vi "Length_8.vi"() -> ()   [LabVIEW 2020]
uses:
  Support/Controls/Cmd_Mouse Popup.ctl
  Support/Controls/Clst_Initialize Input.ctl
  Support/Controls/Clst_Result inspec.ctl
  Support/Controls/Cmd_Var Data IO.ctl
  Variables/Global_Cal Info.vi
  Variables/Global_Cal STD.vi
  Support/Public/Polymorph/Data Class_2D Str.vi
panel:
  in  "기준기 설정":string(combo)
  out "최소범위":string
  out "STD set":string[][](table) caption="○ 기준기 조합 (값)"
  in  "Measured 2":string[][](table)
  in  "표시방식":string(combo)
  out "단위":string
  out "최대범위":string
  in  "Spec 변경":bool
  in  "Random":bool
  out "Resolution":string[][](table) caption="Spec"
  out "Spec":string[][](table)
  out "제목":string
  out "에러 출력":errorcluster
  out "Condition":string[][](table) caption="2. 직선성 시험"
  in  "최소눈금":string(combo)
  in  "Measured":string[][](table) caption="지시편차 (μm)"
  out "Load?":bool
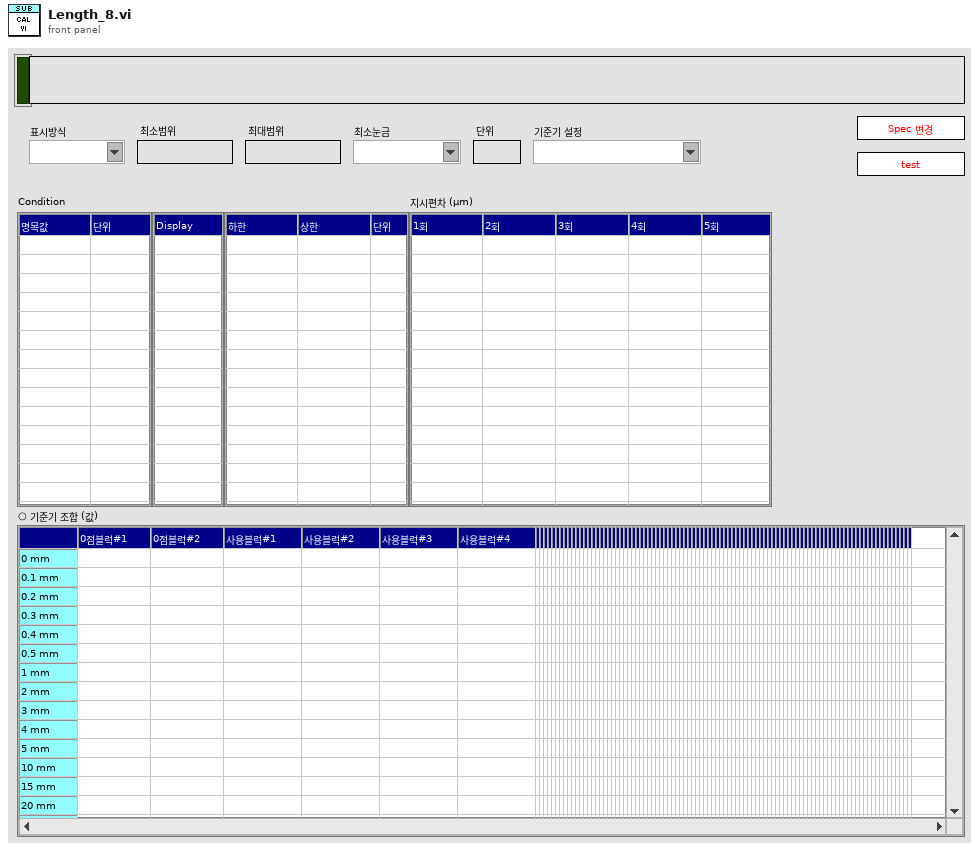
[diagram p1: front panel]
types:
  T1 = typedef "Cmd_Mouse Popup.ctl" = enum16{"활성화", "메뉴선택"}
  T2 = cluster{"Shift":bool, "Ctrl":bool, "Alt":bool, "Cmd":bool, "Opt":bool}
  T3 = typedef "Clst_Initialize Input.ctl" = cluster{"Initialize 1":cluster{"Condition":refnum<vi>[], "Spec":refnum<vi>[], "Measured":refnum<vi>[], "Resolution":refnum<vi>[], "Func_ext":string, "제목":refnum<vi>, "Measured_ADJ":refnum<vi>[]}, "Initialize 2":cluster{"문자열":refnum<vi>[], "콤보박스":refnum<vi>[], "링":refnum<vi>[], "열거형":refnum<vi>[], "테이블":refnum<vi>[], "여러열":refnum<vi>[], "디지털(DBL)":refnum<vi>[], "3D string":refnum<vi>[], "ctrl":refnum<vi>[], "boolean":refnum<vi>[]}}
  T4 = typedef "Clst_Result inspec.ctl" = cluster{"분해능":string, "문자열 1":string, "문자열 2":string, "숫자형 1":i32, "숫자형 2":i32, "숫자형 3":dbl, "문자배열 1D":string[], "문자배열 2D":string[][], "문자배열 3D":string[][][], "문자배열 4D":string[][][][], "불리언 1D":bool[]}
  T5 = typedef "Cmd_Var Data IO.ctl" = enum16{"Condition", "Condition Default", "Condition_Temp", "Resolution", "Resolution Default", "Resolution Old", "Spec", "Spec Default", "Spec Old", "Spec Temp", "Result", "Result2", "Result3", "Result_Temp", "Result_ADJ", "Result_ADJ2", "STD1", "STD2", "STD3", "STD4", "STD5", "STD Temp", "CMC", "CMC Default"}
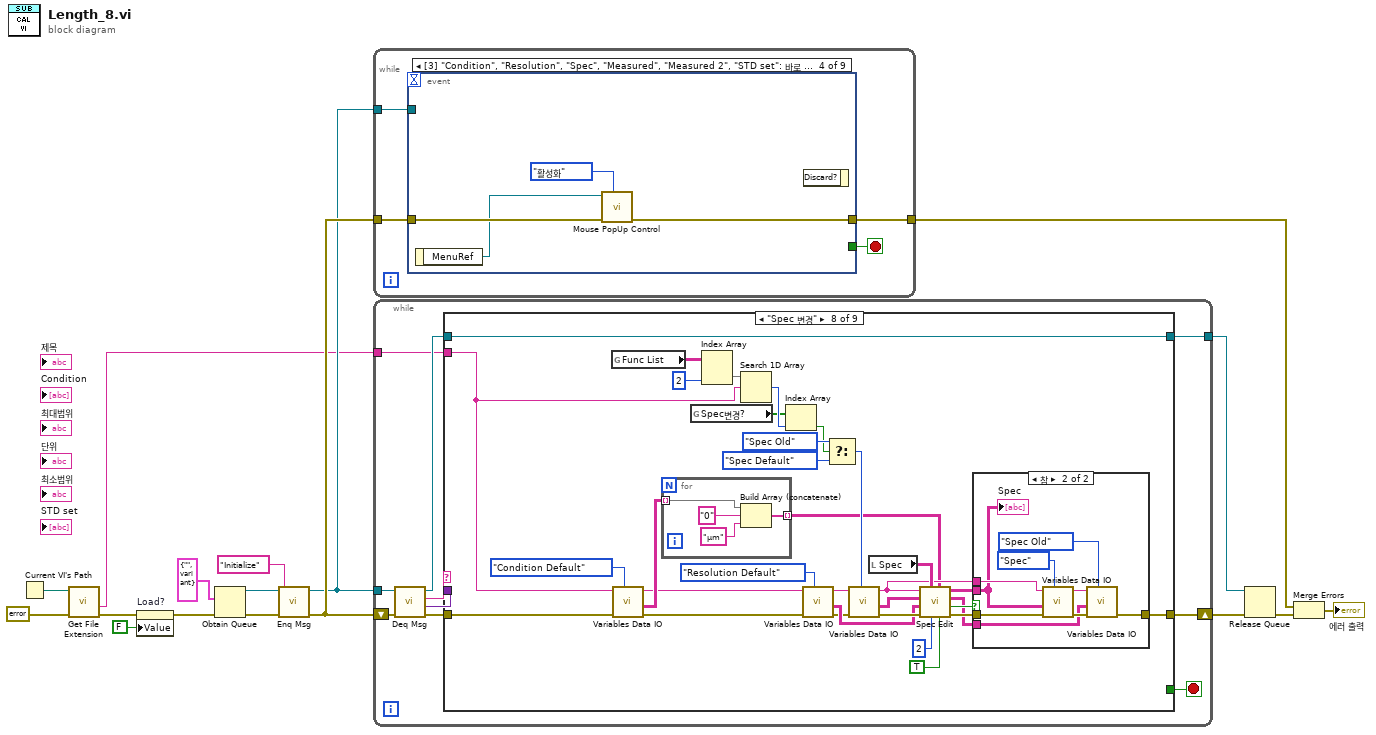
[diagram p0: block diagram]
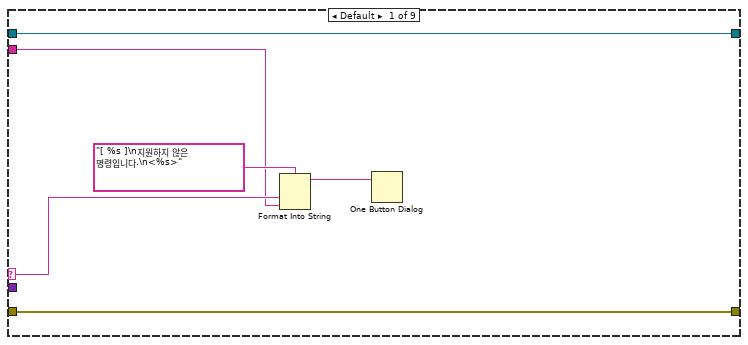
[diagram p2: hidden frame]
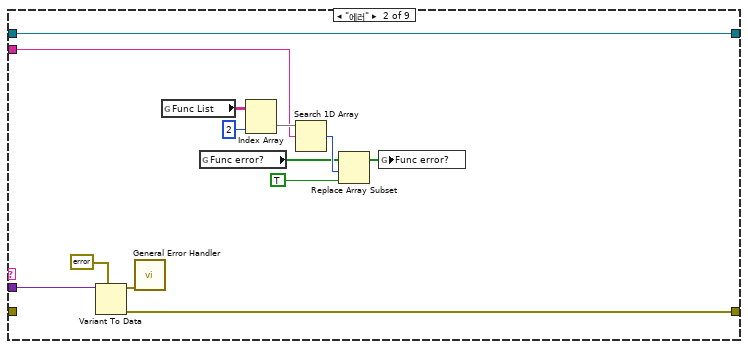
[diagram p3: hidden frame]
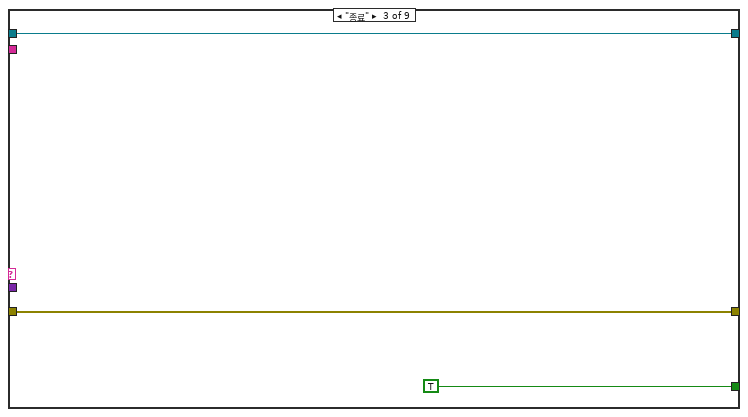
[diagram p4: hidden frame]
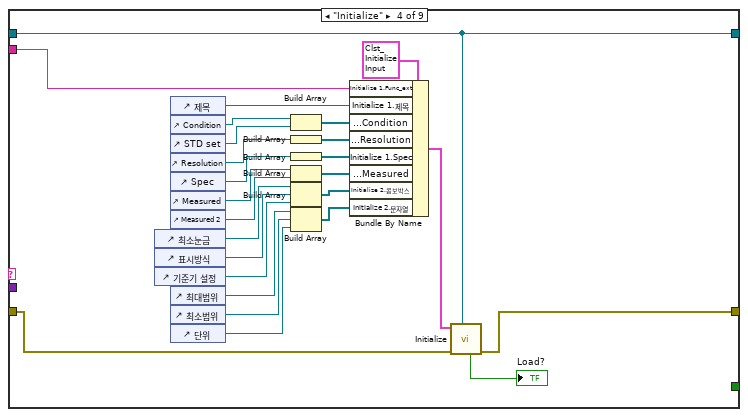
[diagram p5: hidden frame]
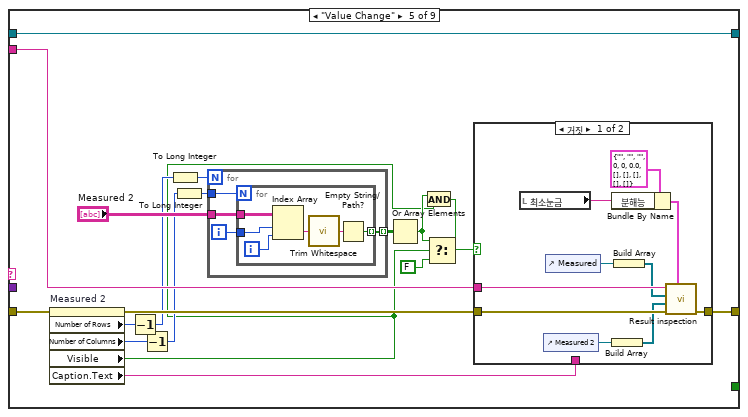
[diagram p6: hidden frame]
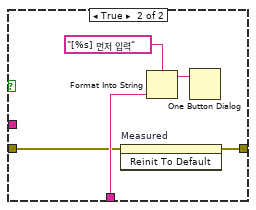
[diagram p7: hidden frame]
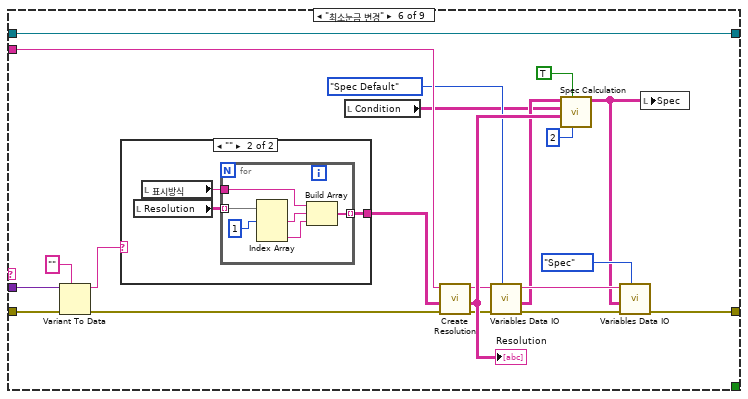
[diagram p8: hidden frame]
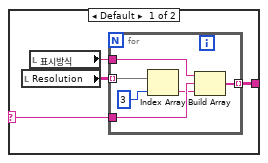
[diagram p9: hidden frame]
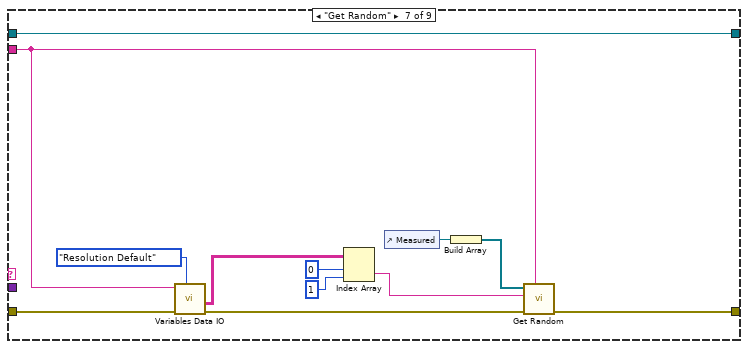
[diagram p10: hidden frame]
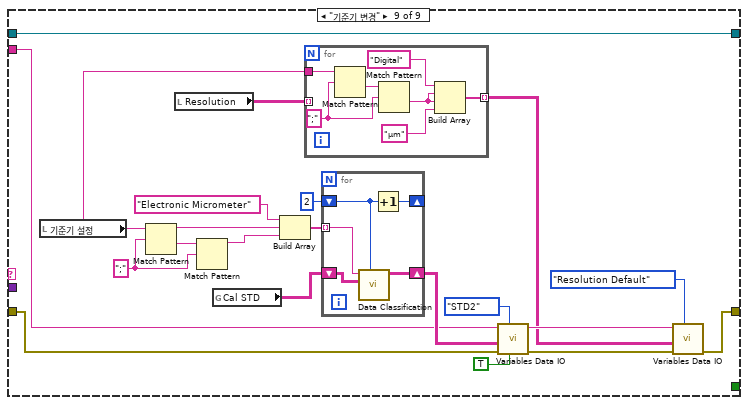
[diagram p12: hidden frame]
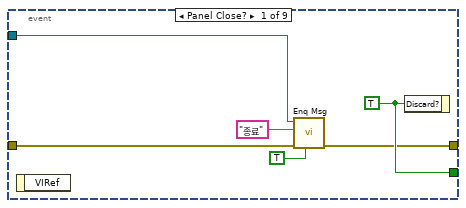
[diagram p13: hidden frame]
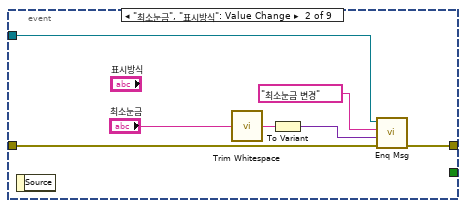
[diagram p14: hidden frame]
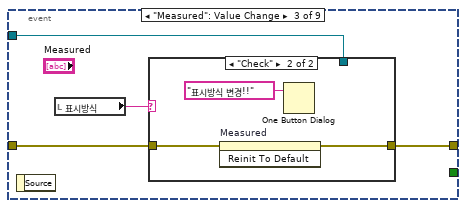
[diagram p15: hidden frame]
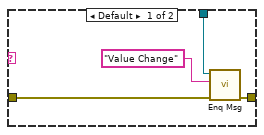
[diagram p16: hidden frame]
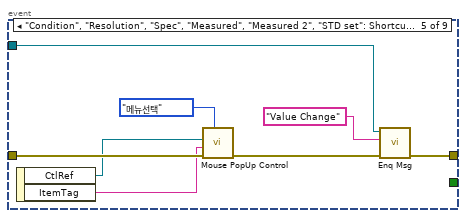
[diagram p17: hidden frame]
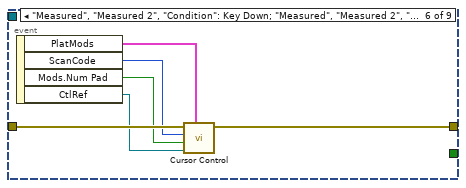
[diagram p18: hidden frame]
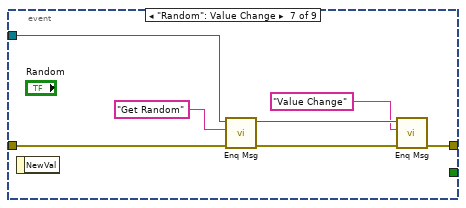
[diagram p19: hidden frame]
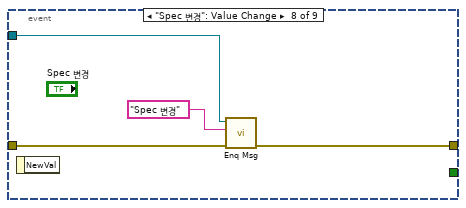
[diagram p20: hidden frame]
diagram:
  n1 = Current VI's Path() -> (path=w5:path)
  n2 = call <vilib>:"Get File Extension.vi"("error in (no error)"=errorcluster {"status"=FALSE, "code"=0, "source"=""} ("에러 상수"), "file"=w5) -> ("error out"=w3:errorcluster, "filename without extension"=w4:string)  [unwired: 5 in, 3 out]
  n3 = property on="Load?" class="Bool (엄격한)"(error in=w3, "Value"=FALSE ("Load?")) -> (error out=w2:errorcluster)  [unwired: 1 in, 1 out]
  n4 = Obtain Queue(element data type=cluster{"메세지":string, "값":variant} {"메세지"="", "값"=variant} ("Message Cluster"), error in (no error)=w2) -> (queue out=w14:refnum<queue>, error out=w16:errorcluster)  [unwired: 3 in, 1 out]
  n5 = call "Enq Msg.vi"("에러 입력(에러 없음)"=w16, "메세지"="Initialize", "큐 입력"=w14) -> ("에러 출력"=w15:errorcluster, "큐 출력"=w12:refnum<queue>)  [unwired: 7 in]
  n6 = while {
    tunnel: w15 -> [w19]
    tunnel: w12 -> [w20]
    tunnel: [w18] -> w9
    stop <- w21 stop-if-true
    n7 = event shown="[3] \"Condition\", \"Resolution\", \"Spec\", \"Measured\", \"Measured 2\", \"STD set\": 바로 가기 메뉴 활성화?" {
      selector: _ -> [_ _ _ _ _ _ _ _ _]
      dyn-events: _ -> [_ _ _ _ _ _ _ _ _]
      timeout: _ -> [_ _ _ _ _ _ _ _ _]
      tunnel: [w27 _ _ _ _ _ _ _ _] -> w21
      tunnel: w20 -> [w25 w33 w38 _ w50 _ w68 w72 w75]
      tunnel: w19 -> [w26 w34 w36 w49 w57 w63 w69 w73 w77]
      tunnel: [w23 w32 w37 w48 w51 w62 w64 w71 w76] -> w18
      event Panel Close? {
        w27 = TRUE ("버림?")
        n8 = event-data() -> ()  [unwired: 1 in, 1 out]
        n9 = call "Enq Msg.vi"("우선순위 메시지?"=TRUE, "에러 입력(에러 없음)"=w26, "메세지"="종료", "큐 입력"=w25) -> ("에러 출력"=w23:errorcluster)  [unwired: 6 in, 1 out]
        n10 = event-data("Discard?"=w27) -> ()  [unwired: 1 in, 1 out]
      }
      event "최소눈금", "표시방식": Value Change {
        n11 = event-data() -> ()  [unwired: 1 in, 1 out]
        n12 = call <vilib>:"Trim Whitespace.vi"("string"="최소눈금") -> ("trimmed string"=w30:string)  [unwired: 1 in]
        n13 = To Variant(anything=w30) -> (Variant=w28:variant)
        n14 = call "Enq Msg.vi"("에러 입력(에러 없음)"=w34, "값"=w28, "메세지"="최소눈금 변경", "큐 입력"=w33) -> ("에러 출력"=w32:errorcluster)  [unwired: 6 in, 1 out]
      }
      event "Measured": Value Change {
        n15 = event-data() -> ()  [unwired: 1 in, 1 out]
        n16 = local read "표시방식"() -> (w35:string)
        n17 = case shown="\"Check\"" w35 {
          tunnel: w38 -> [w42 _]
          tunnel: [w41 w43] -> w37
          tunnel: w36 -> [w40 w44]
          frame Default {
            n18 = call "Enq Msg.vi"("에러 입력(에러 없음)"=w40, "메세지"="Value Change", "큐 입력"=w42) -> ("에러 출력"=w41:errorcluster)  [unwired: 7 in, 1 out]
          }
          frame "Check" {
            n19 = invoke on="Measured" class="Tbl (엄격한)" method="Reinit To Default"(error in=w44) -> (error out=w43:errorcluster)  [unwired: 2 in, 2 out]
            n20 = One Button Dialog(message="표시방식 변경!!" ("메시지")) -> ()  [unwired: 1 in, 1 out]
          }
        }
      }
      event "Condition", "Resolution", "Spec", "Measured", "Measured 2", "STD set": Shortcut Menu Activation? {
        n21 = event-data() -> ("MenuRef"=w47:refnum<k9>)  [unwired: 1 in]
        n22 = call "Mouse PopUp Control.vi"("type"=Cmd_Mouse_Popup."활성화", "error in"=w49, "메뉴 참조"=w47) -> ("error out"=w48:errorcluster)  [unwired: 8 in]
        n23 = event-data() -> ()  [unwired: 2 in, 1 out]
      }
      event "Condition", "Resolution", "Spec", "Measured", "Measured 2", "STD set": Shortcut Menu Selection (User) {
        n24 = event-data() -> ("CtlRef"=w55:refnum<vi>, "ItemTag"=w54:string)  [unwired: 1 in]
        n25 = call "Mouse PopUp Control.vi"("type"=Cmd_Mouse_Popup."메뉴선택", "error in"=w57, "아이템 태그"=w54, "Tbl 참조 번호"=w55) -> ("error out"=w52:errorcluster)  [unwired: 7 in]
        n26 = call "Enq Msg.vi"("에러 입력(에러 없음)"=w52, "메세지"="Value Change", "큐 입력"=w50) -> ("에러 출력"=w51:errorcluster)  [unwired: 7 in, 1 out]
      }
      event "Measured", "Measured 2", "Condition": Key Down; "Measured", "Measured 2", "Condition": Key Repeat {
        n27 = event-data() -> ("PlatMods"=w58:T2, "ScanCode"=w61:i16, "Mods.Num Pad"=w60:bool, "CtlRef"=w59:refnum<vi>)  [unwired: 1 in]
        n28 = call "Cursor Control.vi"("플랫폼 조합키"=w58, "참조"=w59, "Num Pad"=w60, "ScanCode"=w61, "error in"=w63) -> ("error out"=w62:errorcluster)  [unwired: 5 in, 1 out]
      }
      event "Random": Value Change {
        n29 = event-data() -> ()  [unwired: 1 in, 1 out]
        n30 = call "Enq Msg.vi"("에러 입력(에러 없음)"=w69, "메세지"="Get Random", "큐 입력"=w68) -> ("에러 출력"=w67:errorcluster, "큐 출력"=w66:refnum<queue>)  [unwired: 7 in]
        n31 = call "Enq Msg.vi"("에러 입력(에러 없음)"=w67, "메세지"="Value Change", "큐 입력"=w66) -> ("에러 출력"=w64:errorcluster)  [unwired: 7 in, 1 out]
      }
      event "Spec 변경": Value Change {
        n32 = event-data() -> ()  [unwired: 1 in, 1 out]
        n33 = call "Enq Msg.vi"("에러 입력(에러 없음)"=w73, "메세지"="Spec 변경", "큐 입력"=w72) -> ("에러 출력"=w71:errorcluster)  [unwired: 7 in, 1 out]
      }
      event "기준기 설정": Value Change {
        n34 = event-data() -> ()  [unwired: 1 in, 2 out]
        n35 = call "Enq Msg.vi"("에러 입력(에러 없음)"=w77, "메세지"="기준기 변경", "큐 입력"=w75) -> ("에러 출력"=w76:errorcluster)  [unwired: 7 in, 1 out]
      }
    }
  }
  n36 = while {
    shift-right: [w88] -> w11
    shift-left: w15 -> [w87]
    tunnel: w12 -> [w85]
    tunnel: [w80] -> w10
    tunnel: w4 -> [w79]
    stop <- w81 stop-if-true
    n37 = call "Deq Msg.vi"("에러 입력(에러 없음)"=w87, "큐 입력"=w85) -> ("에러 출력"=w86:errorcluster, "값"=w82:variant, "메세지"=w84:string, "큐 출력"=w83:refnum<queue>)  [unwired: 6 in]
    n38 = case shown="\"Spec 변경\"" w84 {
      selector: w84 -> [w90 _ _ _ _ _ _ _ _]
      tunnel: w86 -> [w94 _ w110 w113 w150 w199 w227 w239 w291]
      tunnel: [w94 w104 w110 w127 w153 w192 w228 w259 w286] -> w88
      tunnel: w83 -> [w93 w103 w108 w121 w154 w200 w231 w263 w298]
      tunnel: w82 -> [_ w105 _ _ _ w198 _ _ _]
      tunnel: [_ _ TRUE ("버림?") _ _ _ _ _ _] -> w81
      tunnel: [w93 w103 w108 w121 w154 w200 w231 w263 w298] -> w80
      tunnel: w79 -> [w89 w95 _ w122 w152 w196 w224 w233 w290]
      frame Default {
        n39 = Format Into String(format string="[ %s ]\n지원하지 않은 명령입니다.\n<%s>" ("메시지"), w90, w89) -> (resulting string=w91:string)  [unwired: 2 in, 1 out]
        n40 = One Button Dialog(message=w91) -> ()  [unwired: 1 in, 1 out]
      }
      frame "에러" {
        n41 = Variant To Data(type=errorcluster {"status"=FALSE, "code"=0, "source"=""} ("에러 출력"), Variant=w105) -> (data=w107:errorcluster, error out=w104:errorcluster)  [unwired: 1 in]
        n42 = call <vilib>:"General Error Handler.vi"("error in (no error)"=w107) -> ()  [unwired: 10 in, 5 out]
        n43 = global read "Global_Cal Info.vi" "Func List"() -> (w97:string[][])
        n44 = global read "Global_Cal Info.vi" "Func error?"() -> (w100:bool[])
        n45 = Index Array(array=w97, index (col)=2 ("비활성화된 인덱스 (열)")) -> (element=w98:string[])  [unwired: 1 in]
        n46 = Search 1D Array(1D array=w98, element=w95) -> (index of element=w101:i32)  [unwired: 1 in]
        n47 = Replace Array Subset(array=w100, new element=TRUE ("새 원소/부분배열"), index=w101) -> (w102:bool[])
        n48 = global write "Global_Cal Info.vi" "Func error?"(w102) -> ()
      }
      frame "종료" {
      }
      frame "Initialize" {
        n49 = control-ref of="최소눈금"() -> (w120:refnum<vi>)
        n50 = control-ref of="표시방식"() -> (w130:refnum<vi>)
        n51 = control-ref of="기준기 설정"() -> (w114:refnum<vi>)
        n52 = control-ref of="제목"() -> (w128:refnum<vi>)
        n53 = control-ref of="Condition"() -> (w134:refnum<vi>)
        n54 = control-ref of="STD set"() -> (w112:refnum<vi>)
        n55 = control-ref of="Resolution"() -> (w123:refnum<vi>)
        n56 = control-ref of="Spec"() -> (w126:refnum<vi>)
        n57 = control-ref of="Measured"() -> (w131:refnum<vi>)
        n58 = control-ref of="Measured 2"() -> (w116:refnum<vi>)
        n59 = control-ref of="최대범위"() -> (w115:refnum<vi>)
        n60 = control-ref of="최소범위"() -> (w117:refnum<vi>)
        n61 = control-ref of="단위"() -> (w119:refnum<vi>)
        n62 = Build Array(w134, w112) -> (w133:refnum<vi>[])
        n63 = Build Array(w123) -> (w124:refnum<vi>[])
        n64 = Build Array(w126) -> (w125:refnum<vi>[])
        n65 = Build Array(w131, w116) -> (w132:refnum<vi>[])
        n66 = Build Array(w120, w130, w114) -> (w129:refnum<vi>[])
        n67 = Build Array(w115, w117, w119) -> (w118:refnum<vi>[])
        n68 = Bundle By Name(cluster=T3 {"Initialize 1"={"Condition"=[], "Spec"=[], "Measured"=[], "Resolution"=[], "Func_ext"="", "제목"=refnum, "Measured_ADJ"=[]}, "Initialize 2"={"문자열"=[], "콤보박스"=[], "링"=[], "열거형"=[], "테이블"=[], "여러열"=[], "디지털(DBL)"=[], "3D string"=[], "ctrl"=[], "boolean"=[]}} ("입력 클러스터"), "Initialize 1.Func_ext"=w122, "Initialize 1.제목"=w128, "Initialize 1.Condition"=w133, "Initialize 1.Resolution"=w124, "Initialize 1.Spec"=w125, "Initialize 1.Measured"=w132, "Initialize 2.콤보박스"=w129, "Initialize 2.문자열"=w118) -> (w135:T3)
        n69 = call "Initialize.vi"("큐 입력"=w121, "error in"=w113, "입력 클러스터"=w135) -> ("error out"=w127:errorcluster, "Load?"=→"Load?":bool)  [unwired: 5 in, 2 out]
      }
      frame "Value Change" {
        n70 = property on="Measured 2" class="Tbl (엄격한)"(error in=w150) -> (error out=w149:errorcluster, "Number of Rows"=w151:u32, "Number of Columns"=w144:u32, "Visible"=w138:bool, "Caption.Text"=w147:string)  [unwired: 1 in, 1 out]
        n71 = Decrement(x=w151) -> (x-1=w145:u32)
        n72 = Decrement(x=w144) -> (x-1=w143:u32)
        n73 = To Long Integer(number=w145) -> (32bit integer=w141:i32)
        n74 = To Long Integer(number=w143) -> (32bit integer=w142:i32)
        n75 = for {
          N: w141 -> [_]
          tunnel: "Measured 2" -> [w157]
          tunnel: w142 -> [w158]
          tunnel: [w156] -> w140 mode=indexing
          i -> [w155]
          n76 = for {
            N: w158 -> [_]
            tunnel: w157 -> [w162]
            tunnel: [w163] -> w156 mode=indexing
            tunnel: w155 -> [w160]
            i -> [w159]
            n77 = Index Array(array=w162, index (row)=w160, index (col)=w159) -> (element=w161:string)
            n78 = call <vilib>:"Trim Whitespace.vi"("string"=w161) -> ("trimmed string"=w164:string)  [unwired: 1 in]
            n79 = Empty String/Path?(string/path=w164) -> (empty?=w163:bool)
          }
        }
        n80 = Or Array Elements(Boolean array=w140) -> (logical OR=w139:bool)
        n81 = And(x=w139, y=w138) -> (x .and. y?=w137:bool)
        n82 = Select(t=w139, s=w138, f=FALSE) -> ()  [unwired: 1 out]
        n83 = case shown="거짓" w137 {
          tunnel: [w174 w175] -> w153
          tunnel: w152 -> [w173 _]
          tunnel: w149 -> [w167 w176]
          tunnel: w147 -> [_ w179]
          frame False {
            n84 = local read "최소눈금"() -> (w169:string)
            n85 = control-ref of="Measured 2"() -> (w166:refnum<vi>)
            n86 = control-ref of="Measured"() -> (w172:refnum<vi>)
            n87 = Bundle By Name(cluster=T4 {"분해능"="", "문자열 1"="", "문자열 2"="", "숫자형 1"=0, "숫자형 2"=0, "숫자형 3"=0.0, "문자배열 1D"=[], "문자배열 2D"=[], "문자배열 3D"=[], "문자배열 4D"=[], "불리언 1D"=[]} ("입력 클러스터"), "분해능"=w169) -> (w168:T4)
            n88 = Build Array(w166) -> (w165:refnum<vi>[])
            n89 = Build Array(w172) -> (w171:refnum<vi>[])
            n90 = call "Result inspection.vi"("입력 클러스터"=w168, "error in"=w167, "Ref. Data (excluded)"=w165, "Ref. Data (Inspection)"=w171, "Func ext"=w173) -> ("error out"=w174:errorcluster)  [unwired: 3 in, 3 out]
          }
          frame True {
            n91 = invoke on="Measured" class="Tbl (엄격한)" method="Reinit To Default"(error in=w176) -> (error out=w175:errorcluster)  [unwired: 2 in, 2 out]
            n92 = Format Into String(format string="[%s] 먼저 입력" ("포맷 문자열"), w179) -> (resulting string=w177:string)  [unwired: 2 in, 1 out]
            n93 = One Button Dialog(message=w177) -> ()  [unwired: 1 in, 1 out]
          }
        }
      }
      frame "최소눈금 변경" {
        n94 = Variant To Data(error in=w199, type="", Variant=w198) -> (data=w182:string, error out=w185:errorcluster)
        n95 = case shown="\"\"" w182 {
          selector: w182 -> [w201 _]
          tunnel: [w204 w213] -> w184
          frame Default {
            n96 = local read "Resolution"() -> (w203:string[][])
            n97 = local read "표시방식"() -> (w202:string)
            n98 = for {
              tunnel: w203 -> [w210] mode=indexing
              tunnel: w201 -> [w209]
              tunnel: [w207] -> w204 mode=indexing
              tunnel: w202 -> [w206]
              n99 = Index Array(array=w210, index=3 ("인덱스")) -> (element=w208:string)
              n100 = Build Array(w206, w209, w208) -> (w207:string[])
            }
          }
          frame "" {
            n101 = local read "Resolution"() -> (w212:string[][])
            n102 = local read "표시방식"() -> (w211:string)
            n103 = for {
              tunnel: w212 -> [w219] mode=indexing
              tunnel: [w218] -> w213 mode=indexing
              tunnel: w211 -> [w217]
              n104 = Index Array(array=w219, index #1=1 ("인덱스")) -> (element #1=w215:string, element #3=w214:string)  [unwired: 2 in, 1 out]
              n105 = Build Array(w217, w215, w214) -> (w218:string[])
            }
          }
        }
        n106 = local read "Condition"() -> (w183:string[][])
        n107 = call "Create Resolution.vi"("에러 입력(에러 없음)"=w185, "Resolution"=w184, "Func_ext"=w196) -> ("에러 출력"=w190:errorcluster, "Resolution Out"=w193:string[][], "Func_ext 출력"=w188:string)  [unwired: 6 in]
        "Resolution" <- w193
        n108 = call "Variables Data IO.vi"("Select"=Cmd_Var_Data_IO."Spec Default", "error in"=w190, "Func_ext"=w188) -> ("error out"=w189:errorcluster, "Data Out"=w186:string[][], "Func_ext Out"=w187:string)  [unwired: 6 in]
        n109 = call "Spec Calculation.vi"("기준값 열번호"=2 ("열번호(기준값)"), "0기준?"=TRUE, "Resolution"=w193, "Condition in"=w183, "Spec Default"=w186) -> ("Spec out"=w181:string[][])  [unwired: 5 in, 1 out]
        n110 = call "Variables Data IO.vi"("Select"=Cmd_Var_Data_IO."Spec", "error in"=w189, "Data In"=w181, "Func_ext"=w187) -> ("error out"=w192:errorcluster)  [unwired: 5 in, 2 out]
        n111 = local write "Spec"(w181) -> ()
      }
      frame "Get Random" {
        n112 = call "Variables Data IO.vi"("Select"=Cmd_Var_Data_IO."Resolution Default", "error in"=w227, "Func_ext"=w224) -> ("error out"=w226:errorcluster, "Data Out"=w223:string[][])  [unwired: 6 in, 1 out]
        n113 = Index Array(array=w223, index (row)=0 ("인덱스 (행)"), index (col)=1 ("비활성화된 인덱스 (열)")) -> (element=w220:string)
        n114 = control-ref of="Measured"() -> (w230:refnum<vi>)
        n115 = Build Array(w230) -> (w229:refnum<vi>[])
        n116 = call "Get Random.vi"("Func_Ext"=w224, "에러 입력"=w226, "분해능"=w220, "Meas"=w229) -> ("에러 출력"=w228:errorcluster)  [unwired: 6 in, 1 out]
      }
      frame "Spec 변경" {
        n117 = global read "Global_Cal Info.vi" "Func List"() -> (w247:string[][])
        n118 = call "Variables Data IO.vi"("Select"=Cmd_Var_Data_IO."Condition Default", "error in"=w239, "Func_ext"=w233) -> ("error out"=w238:errorcluster, "Data Out"=w237:string[][], "Func_ext Out"=w234:string)  [unwired: 6 in]
        n119 = for {
          tunnel: [w267] -> w236 mode=indexing
          tunnel: w237 -> [w264] mode=indexing
          n120 = Build Array (concatenate)(w264, "0" ("원소"), "μm" ("원소")) -> (w267:string[])
        }
        n121 = global read "Global_Cal Info.vi" "Spec변경?"() -> (w243:bool[])
        n122 = Index Array(array=w247, index (col)=2 ("비활성화된 인덱스 (열)")) -> (element=w245:string[])  [unwired: 1 in]
        n123 = Search 1D Array(1D array=w245, element=w233) -> (index of element=w244:i32)  [unwired: 1 in]
        n124 = Index Array(array=w243, index=w244) -> (element=w248:bool)
        n125 = call "Variables Data IO.vi"("Select"=Cmd_Var_Data_IO."Resolution Default", "error in"=w238, "Func_ext"=w234) -> ("error out"=w240:errorcluster, "Data Out"=w251:string[][], "Func_ext Out"=w235:string)  [unwired: 6 in]
        n126 = Select(t=Cmd_Var_Data_IO."Spec Old" ("Select"), s=w248, f=Cmd_Var_Data_IO."Spec Default" ("Select")) -> (s? t:f=w242:T5)
        n127 = call "Variables Data IO.vi"("Select"=w242, "error in"=w240, "Func_ext"=w235) -> ("error out"=w258:errorcluster, "Data Out"=w252:string[][], "Func_ext Out"=w253:string)  [unwired: 6 in]
        n128 = local read "Spec"() -> (w254:string[][])
        n129 = call "Spec Edit.vi"("0기준?"=TRUE, "Condition"=w236, "열번호(기준값)"=2, "Spec Value"=w254, "에러 입력(에러 없음)"=w258, "Resolution"=w251, "Spec Default"=w252, "Func_ext"=w253) -> ("에러 출력"=w260:errorcluster, "변경?"=w261:bool, "Spec Default out"=w256:string[][], "Spec 출력"=w262:string[][])
        n130 = case shown="참" w261 {
          tunnel: w262 -> [_ w274]
          tunnel: w260 -> [w268 w277]
          tunnel: [w268 w272] -> w259
          tunnel: w253 -> [_ w275]
          tunnel: w256 -> [_ w270]
          frame False {
          }
          frame True {
            n131 = call "Variables Data IO.vi"("Select"=Cmd_Var_Data_IO."Spec", "error in"=w277, "Data In"=w274, "Func_ext"=w275) -> ("error out"=w273:errorcluster, "Func_ext Out"=w271:string)  [unwired: 5 in, 1 out]
            n132 = call "Variables Data IO.vi"("Select"=Cmd_Var_Data_IO."Spec Old", "error in"=w273, "Data In"=w270, "Func_ext"=w271) -> ("error out"=w272:errorcluster)  [unwired: 5 in, 2 out]
            "Spec" <- w274
          }
        }
      }
      frame "기준기 변경" {
        w281 = ";" ("정규식")
        n133 = local read "기준기 설정"() -> (w280:string)
        n134 = Match Pattern(string=w280, regular expression=w281) -> (before substring=w297:string, after substring=w283:string)  [unwired: 1 in, 2 out]
        n135 = local read "Resolution"() -> (w279:string[][])
        n136 = Match Pattern(string=w283, regular expression=w281) -> (before substring=w282:string)  [unwired: 1 in, 3 out]
        n137 = global read "Global_Cal STD.vi" "Cal STD"() -> (w288:string[][])
        n138 = Build Array("Electronic Micrometer", w297, w282) -> (w289:string[])
        n139 = for {
          tunnel: w280 -> [w300]
          tunnel: [w305] -> w278 mode=indexing
          tunnel: w279 -> [_] mode=indexing
          w301 = ";" ("정규식")
          n140 = Match Pattern(string=w300, regular expression=w301) -> (after substring=w302:string)  [unwired: 1 in, 3 out]
          n141 = Match Pattern(string=w302, regular expression=w301) -> (after substring=w299:string)  [unwired: 1 in, 3 out]
          n142 = Build Array("Digital" ("원소"), w299, w299, "μm" ("원소")) -> (w305:string[])
        }
        n143 = for {
          shift-right: [w309] -> w295
          shift-left: w288 -> [w310]
          tunnel: w289 -> [w308] mode=indexing
          shift-right: [w306] -> _
          shift-left: 2 ("비활성화된 인덱스 (열)") -> [w307]
          n144 = call-poly "Data Classification.vi"("인덱스"=w307, "DATA 입력"=w310, "검색 문자열"=w308) -> ("DATA 출력"=w309:string[][])  [unwired: 4 in, 4 out]
          n145 = Increment(x=w307) -> (x+1=w306:i32)
        }
        n146 = call "Variables Data IO.vi"("Write blank data ?(F)"=TRUE ("Write blank data ?(T)"), "Select"=Cmd_Var_Data_IO."STD2", "error in"=w291, "Data In"=w295, "Func_ext"=w290) -> ("error out"=w287:errorcluster, "Func_ext Out"=w285:string)  [unwired: 4 in, 1 out]
        n147 = call "Variables Data IO.vi"("Select"=Cmd_Var_Data_IO."Resolution Default", "error in"=w287, "Data In"=w278, "Func_ext"=w285) -> ("error out"=w286:errorcluster)  [unwired: 5 in, 2 out]
      }
    }
  }
  n148 = Release Queue(queue=w10, error in (no error)=w11) -> (error out=w8:errorcluster)  [unwired: 1 in, 2 out]
  n149 = Merge Errors(w9, w8) -> (→"에러 출력":errorcluster)
